vi "Read Activation Type.vi"(8 "error in (no error)":errorcluster, 11 "Macro in":refnum<class "Macro.lvclass">) -> (0 "error out":errorcluster, 2 "Activation Type":enum32{"Hotkey", "Automatic"}(ring), 3 "Macro out":refnum<class "Macro.lvclass">)   [LabVIEW 2020, in "MacroAssert.lvlib" / "Macro.lvclass"]
uses:
  Macro.lvclass
  Macro.lvclass/Macro.ctl
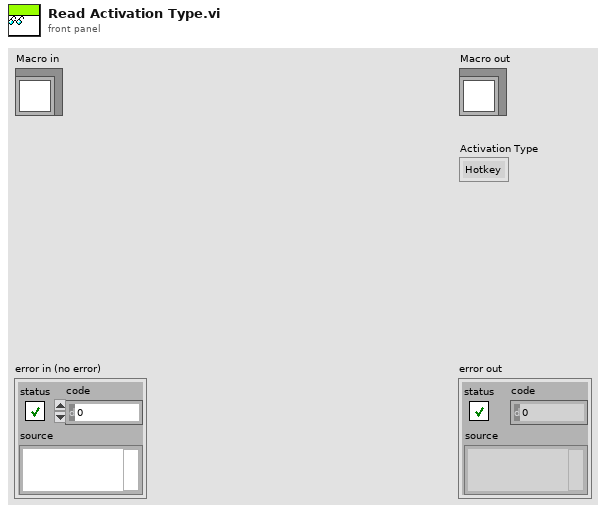
[diagram p1: front panel]
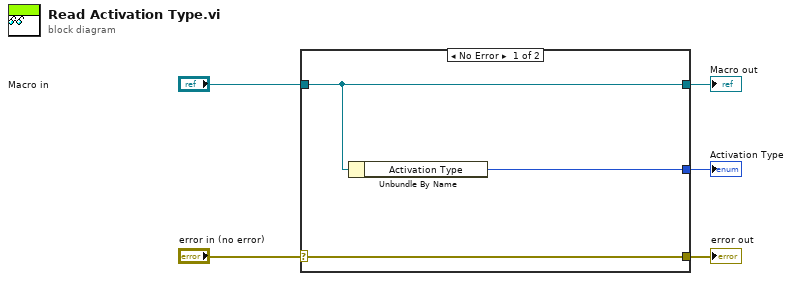
[diagram p0: block diagram]
diagram:
  n1 = case shown="No Error" "error in (no error)" {
    selector: "error in (no error)" -> [w8 w9]
    tunnel: [w8 w9] -> w4
    tunnel: [w7 w10] -> w2
    tunnel: "Macro in" -> [w7 w10]
    tunnel: [w6 _] -> w1
    frame No Error {
      n2 = Unbundle By Name(w7) -> ("Activation Type"=w6:enum32{"Hotkey", "Automatic"})
    }
    frame Error {
    }
  }
  "error out" <- w4
  "Macro out" <- w2
  "Activation Type" <- w1
